vi "Encoder Time Between Counts.vi"(3 "The Encoder Changed":bool, 4 "Ticks between Previous two Encoder Counts (n-1)":u32, 5 "Tick Count at Previous Encoder Count (n-1)":u32, 6 "Current Tick Count":u32) -> (0 "Ticks between Previous two Encoder Counts (n)":u32, 1 "Tick Count at Previous Encoder Count (n)":u32, 2 "Encoder Delta (ticks)":u32)   [LabVIEW 2009]
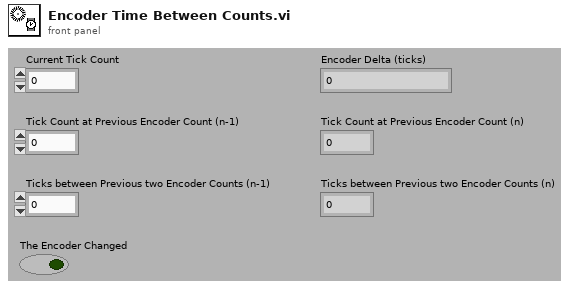
[diagram p1: front panel]
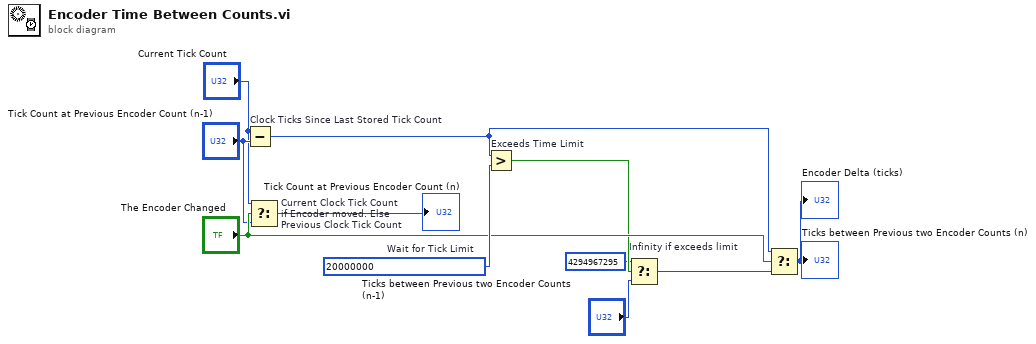
[diagram p0: block diagram]
diagram:
  w11 = u32 20000000  # Wait for Tick Limit
  n1 = Subtract "Clock Ticks Since Last Stored Tick Count"(x="Current Tick Count", y="Tick Count at Previous Encoder Count (n-1)") -> (x-y=w4:u32)
  n2 = Select "Current Clock Tick Count\nif Encoder moved. Else\nPrevious Clock Tick Count"(t="Current Tick Count", s="The Encoder Changed", f="Tick Count at Previous Encoder Count (n-1)") -> (s? t:f=→"Tick Count at Previous Encoder Count (n)":u32)
  n3 = Greater? "Exceeds Time Limit"(x=w4, y=w11) -> (0:w2:bool)
  n4 = Select "Infinity if exceeds limit"(t=u32 4294967295, s=w2, f="Ticks between Previous two Encoder Counts (n-1)") -> (s? t:f=w5:u32)
  n5 = Select(t=w4, s="The Encoder Changed", f=w5) -> (s? t:f=→"Encoder Delta (ticks)" →"Ticks between Previous two Encoder Counts (n)":u32)
